vi "創造圖片(1D).vi"(8 "error In":errorcluster, 10 "影像數量":i32=1, 11 "Image Name":string="Source") -> (0 "error out":errorcluster, 1 "ImageOutNameArray":string[](array[string]), 3 "Image1DArray":T1[](array[typedef]))   [LabVIEW 2015]
uses:
  <vilib>/vision/Image Controls.llb/IMAQ Image.ctl
  Image action.ctl
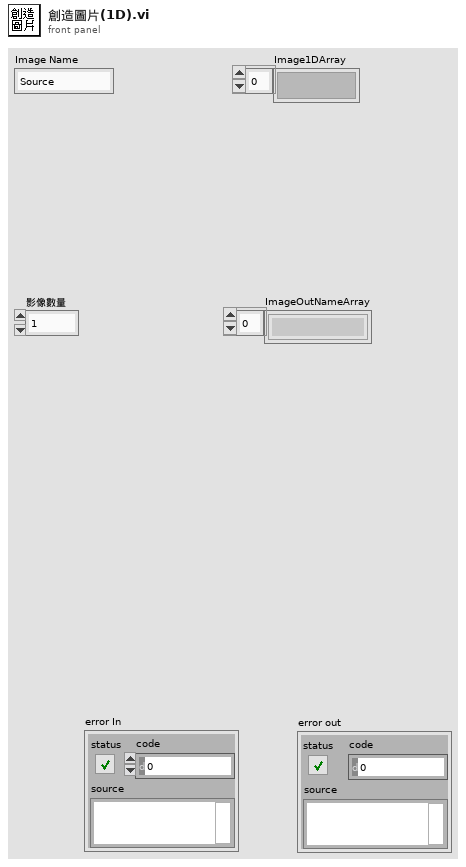
[diagram p1: front panel]
types:
  T1 = typedef "IMAQ Image.ctl" = refnum<image>
  T2 = typedef "Image action.ctl" = enum16{"初始化", "創造記憶體", "寫入圖片", "讀取圖片", "刪除圖片", "等待"}
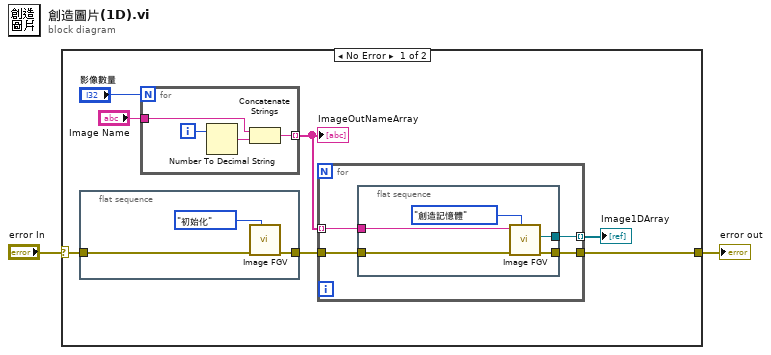
[diagram p0: block diagram]
diagram:
  n1 = case shown="No Error" "error In" {
    selector: "error In" -> [w7 w26]
    tunnel: [w8 w26] -> w2
    frame No Error {
      n2 = flat-sequence {
        tunnel: [w24] -> w6
        tunnel: w7 -> [w23]
        frame #0 {
          n3 = call "Image FGV.vi"("Image action"=Image_action."初始化", "error in (no error)"=w23) -> ("error out"=w24:errorcluster)  [unwired: 8 in, 1 out]
        }
      }
      n4 = for {
        N: "影像數量" -> [_]
        tunnel: "Image Name" -> [w12]
        tunnel: [w10] -> w4 mode=indexing
        i -> [w13]
        n5 = Number To Decimal String(number=w13) -> (decimal integer string=w11:string)  [unwired: 1 in]
        n6 = Concatenate Strings(w12, w11) -> (w10:string)
      }
      "ImageOutNameArray" <- w4
      n7 = for {
        tunnel: w6 -> [w17]
        tunnel: w4 -> [w16] mode=indexing
        tunnel: [w15] -> w8
        tunnel: [w14] -> w9 mode=indexing
        n8 = flat-sequence {
          tunnel: w17 -> [w21]
          tunnel: w16 -> [w20]
          tunnel: [w19] -> w15
          tunnel: [w18] -> w14
          frame #0 {
            n9 = call "Image FGV.vi"("Image action"=Image_action."創造記憶體", "error in (no error)"=w21, "圖片名稱"=w20) -> ("error out"=w19:errorcluster, "Image Out"=w18:T1)  [unwired: 7 in]
          }
        }
      }
      "Image1DArray" <- w9
    }
    frame Error {
    }
  }
  "error out" <- w2
